vi "TestValueReferenceTransport_NoWrite_ReturnError.vi"(8 "error in (no error)":errorcluster, 11 "TestCase in":refnum<class "TestTransport.lvclass">) -> (0 "error out":errorcluster, 3 "TestCase out":refnum<class "TestTransport.lvclass">)   [LabVIEW 2015, in "Transport.lvlib" / "TestTransport.lvclass"]
uses:
  TestTransport.lvclass
  ValueReferenceTransport/ValueReferenceTransport.lvclass/ValueReferenceTransport.ctl
  <vilib>/Utility/error.llb/Error Cluster From Error Code.vi
  ValueReferenceTransport/ValueReferenceTransport.lvclass
panel:
  out "Read Error":errorcluster
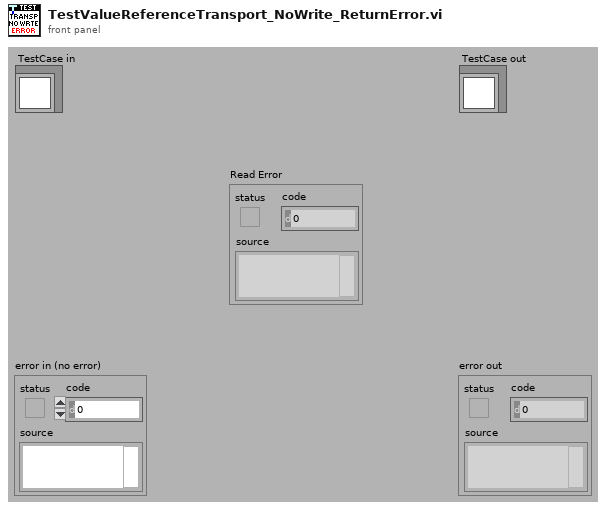
[diagram p1: front panel]
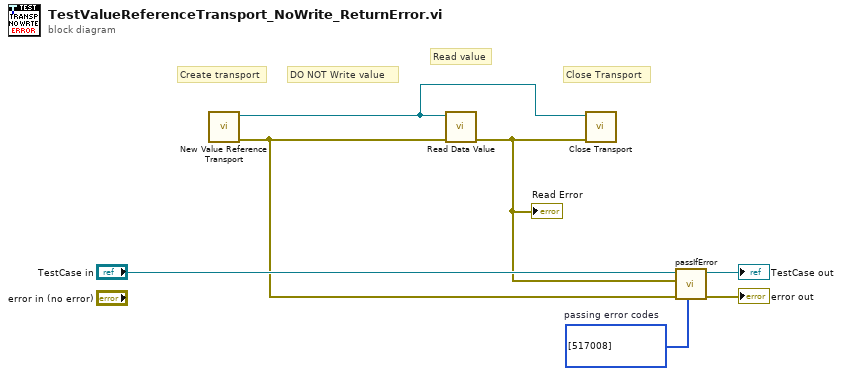
[diagram p0: block diagram]
diagram:
  w1 = i32[] [517008]  # passing error codes
  # "Close Transport"
  # "Create transport"
  # "DO NOT Write value"
  # "Read value"
  n1 = call "New Value Reference Transport.vi"() -> ("error out"=w2:errorcluster, "ValueReferenceTransport"=w4:refnum<class "ValueReferenceTransport.lvclass">)  [unwired: 10 in]
  n2 = call "Read Data Value.vi"("error in (no error)"=w2, "ValueReferenceTransport In"=w4) -> ("error out"=w3:errorcluster)  [unwired: 7 in, 2 out]
  "Read Error" <- w3
  n3 = call-dynamic "Close Transport.vi"("error in (no error)"=w3, "ValueReferenceTransport in"=w4) -> ()  [unwired: 9 in, 1 out]
  n4 = call-dynamic "passIfError.vi"("passing error codes (default = any error code)"=w1, "error in (no error)"=w2, "error"=w3, "TestCase in"="TestCase in") -> ("error out"=→"error out":errorcluster, "TestCase out"=→"TestCase out":refnum<class "TestTransport.lvclass">)  [unwired: 6 in]
